vi "CloseRef.vi"(8 "error in (no error)":errorcluster, 11 "Add in":refnum<class "Add.lvclass">) -> (0 "error out":errorcluster, 3 "Add out":refnum<class "Add.lvclass">)   [LabVIEW 2023, in "Add.lvclass"]
uses:
  Add.lvclass
  Add.lvclass/Add.ctl
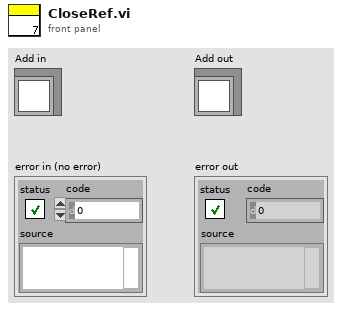
[diagram p1: front panel]
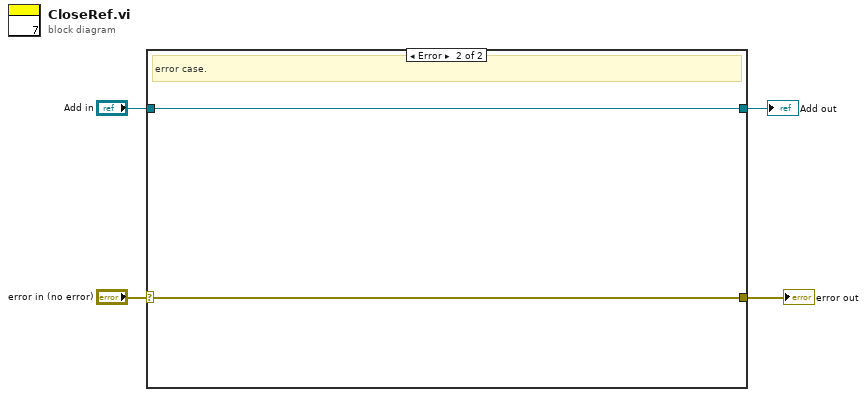
[diagram p0: block diagram]
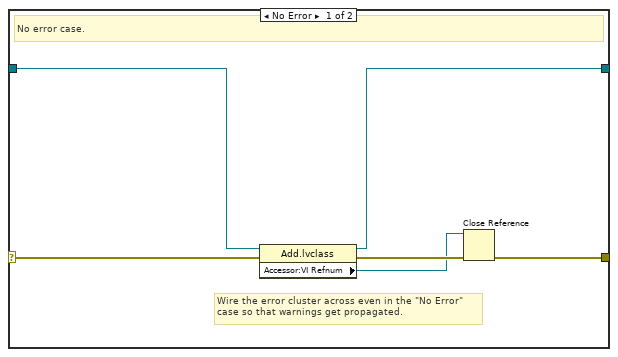
[diagram p2: hidden frame]
diagram:
  n1 = case shown="Error" "error in (no error)" {
    selector: "error in (no error)" -> [w10 w12]
    tunnel: [w7 w12] -> w3
    tunnel: [w5 w11] -> w1
    tunnel: "Add in" -> [w8 w11]
    frame No Error {
      # "Wire the error cluster across even in the \"No Error\"\ncase so that warnings get propagated."
      # "No error case."
      n2 = property class="Add.lvclass"(reference=w8, error in=w10) -> (reference out=w5:refnum<class "Add.lvclass">, error out=w9:errorcluster, "Accessor:VI Refnum"=w6:refnum<vi>)
      n3 = Close Reference(reference=w6, error in (no error)=w9) -> (error out=w7:errorcluster)
    }
    frame Error {
      # "error case."
    }
  }
  "error out" <- w3
  "Add out" <- w1
